vi "qVMA.vi"(0 "System no.":i32=1 min=1 max=4 step=1, 2 "Axes to query":string[](array[string]), 3 "All axes?":bool, 4 "Axis identifier?":bool=TRUE, 5 "error in":errorcluster) -> (14 "Upper PZT limit (V)":dbl[](array[numeric]) format="%.6f", 15 "Channels to query out":string[](array[string]), 19 "error out":errorcluster)   [LabVIEW 2026]
doc: "Returns upper PZT voltage limit for queried axes / piezo channels.\n\nE-516: If All axes = TRUE, then Axis identifier must be TRUE\n\nE-517, E-755: Axes to query are piezo channel numbers. If All axes? = TRUE, then Axis identifier? must be FALSE.\n\nE-761: If All axes = TRUE, then Axis identifier must be FALSE. Axes to query are piezo numbers to query, which can be 1 to 4."
panel:
  # "Returns upper PZT voltage limit of queried axes / piezo channels."
  # "If all axes: use"
  # "Query"
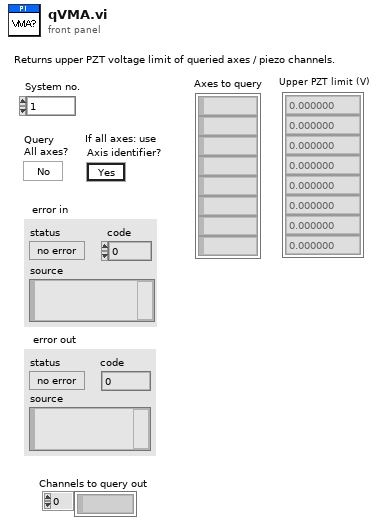
[diagram p1: front panel]
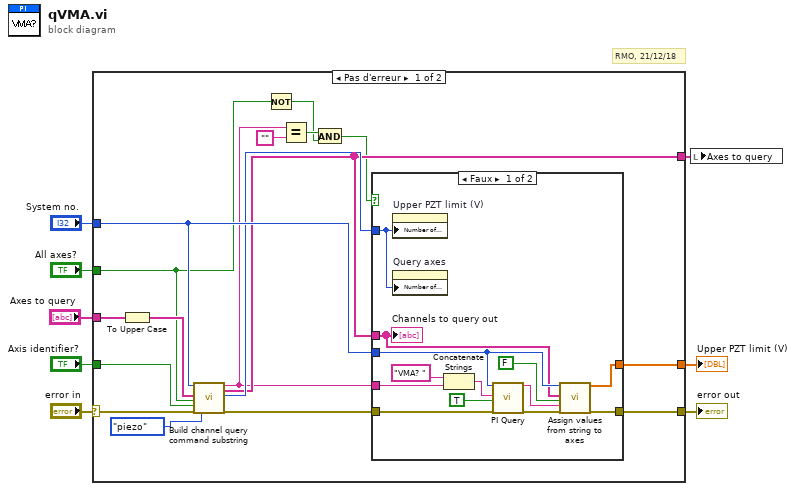
[diagram p0: block diagram]
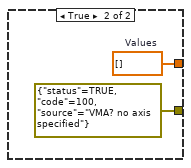
[diagram p2: hidden frame]
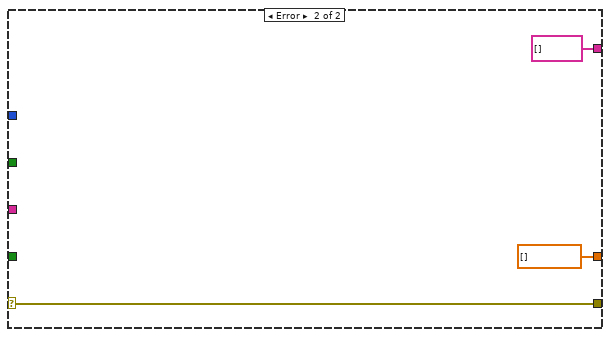
[diagram p3: hidden frame]
diagram:
  # "RMO, 21/12/18"
  n1 = case shown="Pas d'erreur" "error in" {
    selector: "error in" -> [w9 w41]
    tunnel: [w25 dbl[] [] ("Values")] -> w8
    tunnel: "Axes to query" -> [w24 _]
    tunnel: [w11 w41] -> w6
    tunnel: "Axis identifier?" -> [w16 _]
    tunnel: "System no." -> [w19 _]
    tunnel: [w13 string[] [] ("Axes to query out")] -> w3
    tunnel: "All axes?" -> [w17 _]
    frame No Error {
      n2 = To Upper Case(1:w24) -> (0:w18:string[])
      n3 = call "Build channel query command substring.vi"("System no."=w19, "Channels to query in"=w18, "Query\nAll channels?"=w17, "For all channels: use\nChannel identifier?"=w16, "error in"=w9, "Channel type"=enum16{"piezo", "sensor"}."piezo") -> ("Command substring"=w12:string, "Channels to query out"=w13:string[], "Number of rows"=w14:u32, "error out"=w20:errorcluster)  [unwired: 1 in, 9 out]
      n4 = Not(x=w17) -> (.not. x?=w21:bool)
      n5 = Equal?(x=w12, y="" ("x")) -> (x = y?=w22:bool)
      n6 = And(x=w22, y=w21) -> (x .and. y?=w10:bool)
      n7 = case shown="Faux" w10 {
        tunnel: [w35 w39] -> w25
        tunnel: w20 -> [w34 _]
        tunnel: w19 -> [w33 _]
        tunnel: w14 -> [w32 _]
        tunnel: w13 -> [w31 _]
        tunnel: w12 -> [w30 _]
        tunnel: [w28 errorcluster {"status"=TRUE, "code"=100, "source"="VMA? no axis specified"} ("error out")] -> w11
        frame False {
          n8 = property on="Upper PZT limit (V)" class="Tabl (strict)"("Number of Rows"=w32) -> ()  [unwired: 2 in, 2 out]
          n9 = property on="Query axes" class="Tabl (strict)"("Number of Rows"=w32) -> ()  [unwired: 2 in, 2 out]
          n10 = Concatenate Strings("VMA? ", w30) -> (w36:string)
          n11 = call "PI Query.vi"("System no."=w33, "String to send"=w36, "Attach termination char.?"=TRUE ("Attach Linefeed?"), "error in"=w34) -> ("String read"=w26:string, "error out"=w27:errorcluster)  [unwired: 3 in, 11 out]
          n12 = call "Assign values from string to axes.vi"("System no."=w33, "Queried axes"=w31, "All axes queried?"=FALSE, "Input String"=w26, "error in"=w27) -> ("Values"=w35:dbl[], "error out"=w28:errorcluster)  [unwired: 4 in, 9 out]
          "Channels to query out" <- w31
        }
        frame True {
          w39 = dbl[] []  # Values
        }
      }
    }
    frame Error {
    }
  }
  "error out" <- w6
  "Upper PZT limit (V)" <- w8
  n13 = local write "Axes to query"(w3) -> ()
